vi "Reset Axes To Zero.vi"(8 "error in":errorcluster, 10 "axis (def: fine)":enum16{"both", "fine", "coarse"}(ring), 11 "GPIB # (in):def. 6":string="6\n6") -> (0 "error out":errorcluster, 3 "GPIB # (out)":string)   [LabVIEW 2017]
uses:
  mc2mc4.llb/MC2/4  SendCommand.VI
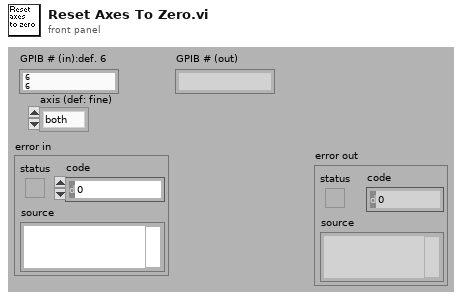
[diagram p1: front panel]
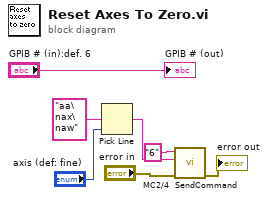
[diagram p0: block diagram]
diagram:
  n1 = Pick Line(multi-line string="aa\nax\naw", line index="axis (def: fine)") -> (output string=w3:string)  [unwired: 1 out]
  n2 = call "MC2/4  SendCommand.VI"("error in (no error)"="error in", "MC2 / MC4 Command"=w3, "GPIB # (in): def.6"="6" ("MC2/MC4 IEEE-488 Address")) -> ("error out"=→"error out":errorcluster)  [unwired: 8 out]
  "GPIB # (out)" <- "GPIB # (in):def. 6"
